vi "RotationOrTorqueConstantConfigUI .vi"() -> (1 "Confirmed?":bool, 3 "RotateOrTorqueConstantConfig":T1)   [LabVIEW 2021]
uses:
  TypeDefs/RotateOrTorqueConstantConfiguration.ctl
panel:
  in  "Duration":dbl caption="Duration (s)"
  in  "Rotation or Torque":string(combo)
  in  "Cancel":bool
  in  "Confirm button":bool
  in  "Constant Value":dbl
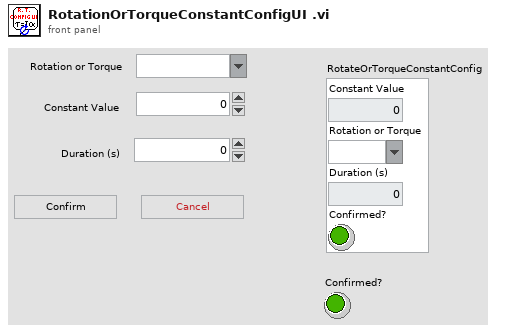
[diagram p1: front panel]
types:
  T1 = typedef "RotateOrTorqueConstantConfiguration.ctl" = cluster{"Constant Value":dbl, "Rotation or Torque":string, "Duration":dbl, "Confirmed?":bool}
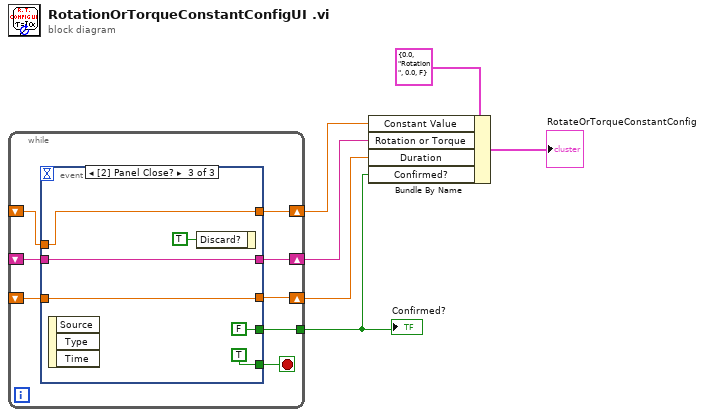
[diagram p0: block diagram]
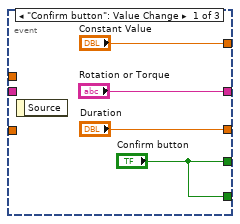
[diagram p2: hidden frame]
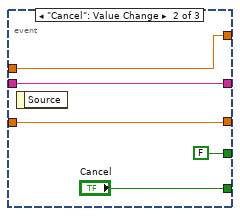
[diagram p3: hidden frame]
diagram:
  n1 = while {
    shift-right: [w14] -> w6
    shift-left: _ -> [w12]
    shift-right: [w13] -> w5
    shift-left: _ -> [w11]
    tunnel: [w10] -> w1
    shift-right: [w8] -> w4
    shift-left: _ -> [w7]
    stop <- w9 stop-if-true
    n2 = event shown="[2] Panel Close?" {
      selector: _ -> [_ _ _]
      dyn-events: _ -> [_ _ _]
      timeout: _ -> [_ _ _]
      tunnel: ["Constant Value" w23 w26] -> w14
      tunnel: ["Rotation or Torque" w21 w25] -> w13
      tunnel: w12 -> [_ w23 w26]
      tunnel: w11 -> [_ w21 w25]
      tunnel: ["Confirm button" FALSE ("Confirm button") FALSE ("Confirm button")] -> w10
      tunnel: ["Confirm button" "Cancel" TRUE ("Cancel")] -> w9
      tunnel: ["Duration" w19 w24] -> w8
      tunnel: w7 -> [_ w19 w24]
      event "Confirm button": Value Change {
        n3 = event-data() -> ()  [unwired: 1 in, 1 out]
      }
      event "Cancel": Value Change {
        n4 = event-data() -> ()  [unwired: 1 in, 1 out]
      }
      event Panel Close? {
        n5 = event-data() -> ()  [unwired: 1 in, 3 out]
        n6 = event-data("Discard?"=TRUE) -> ()  [unwired: 1 in, 1 out]
      }
    }
  }
  "Confirmed?" <- w1
  n7 = Bundle By Name(cluster=T1 {"Constant Value"=0.0, "Rotation or Torque"="Rotation", "Duration"=0.0, "Confirmed?"=FALSE} ("RotateOrTorqueConstantConfig"), "Constant Value"=w6, "Rotation or Torque"=w5, "Duration"=w4, "Confirmed?"=w1) -> (→"RotateOrTorqueConstantConfig":T1)
